vi "General PID Simulator Arduino C code.vi"() -> ()   [LabVIEW 2020]
doc: "This example demonstrates how to simulate a general PID controller."
uses:
  <vilib>/addons/control/pid/NI_PID_pid.lvlib
  <vilib>/addons/control/pid/pid.llb/PID (DBL).vi
panel:
  out "pid_error_integral":dbl=725.9731425642199
  in  "lower limit":dbl
  in  "upper limit":dbl
  in  "Kd":bool=TRUE
  in  "Ki":bool=TRUE
  in  "Kp":bool=TRUE
  in  "loop time[s]":dbl=0.1
  out "PID parameters":dbl[][](graph)=[[30.750899076372775], [7.259731425642199], [0.0]]
  in  "PID type":T1(ring)=enum."Custom C written"
  out "Error":dbl(graph)=1.5375449538186388
  in  "process parameters":T2={"static gain"=2.5, "lag (min)"=18.0, "dead cycles"=0.0, "load %"=40.0, "deadband"=2.0, "noise level %"=0.25, "initial PV"=0.0, "initial PV 2"=0.0}
  out "Manipulated variable":dbl(graph)=38.010630502014976
  in  "SP:":dbl(slide)=88.23529411764706 min=0.0 max=0.0 scale=0.0..100.0
  out "MV:":dbl(slide)=38.010630502014976 scale=-100.0..100.0
  out "PV:":dbl(slide)=86.69774916382842 scale=0.0..100.0
  in  "PID gains":T3={"proportional gain (Kc)"=20.0, "integral time (Ti, min)"=0.01, "derivative time (Td, min)"=0.001} {"derivative time (Td, min)" format="%.3f"; "integral time (Ti, min)" format="%.3f"; "proportional gain (Kc)" format="%.3f"}
  in  "Stop":bool
  out "Process variable and Setpoint":cluster{"initial PV":dbl, "SP:":dbl}(graph)={"initial PV"=86.69774916382842, "SP:"=88.23529411764706}
  # "20,000"
  # "0,008"
  # "0,001"
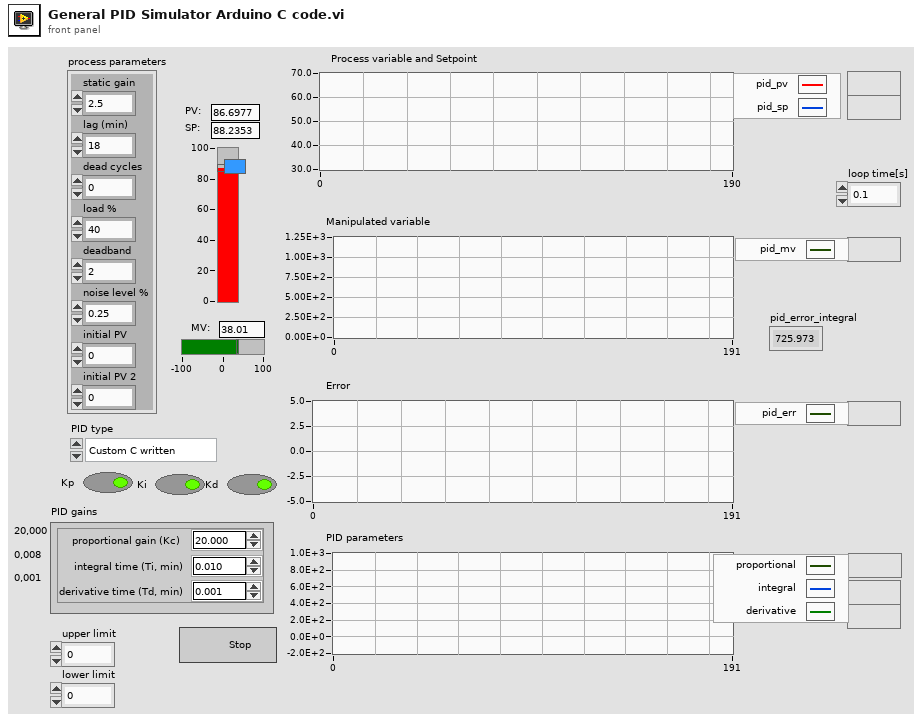
[diagram p1: front panel]
types:
  T1 = enum16{"Official LabVIEW", "Custom LabVIEW", "Custom C written"}
  T2 = cluster{"static gain":dbl, "lag (min)":dbl, "dead cycles":dbl, "load %":dbl, "deadband":dbl, "noise level %":dbl, "initial PV":dbl, "initial PV 2":dbl}
  T3 = cluster{"proportional gain (Kc)":dbl, "integral time (Ti, min)":dbl, "derivative time (Td, min)":dbl}
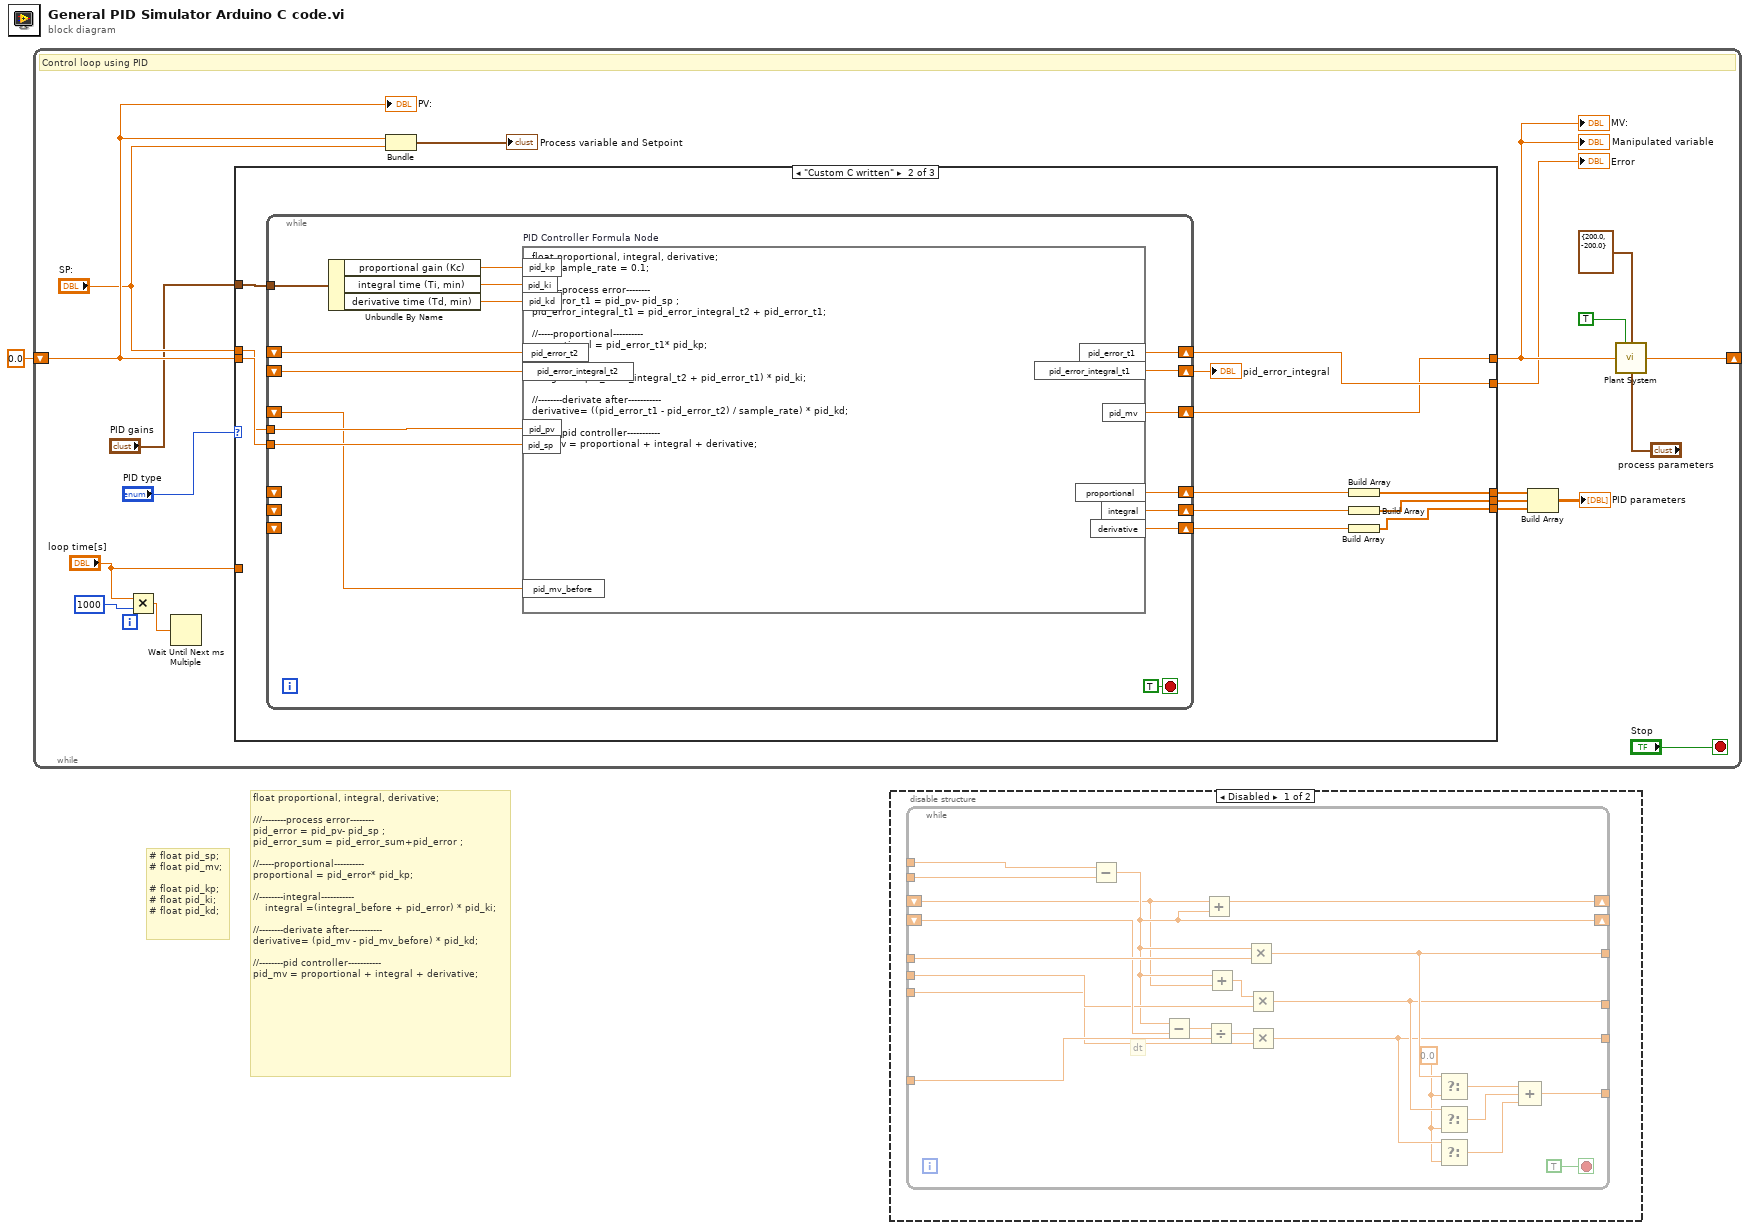
[diagram p0: block diagram]
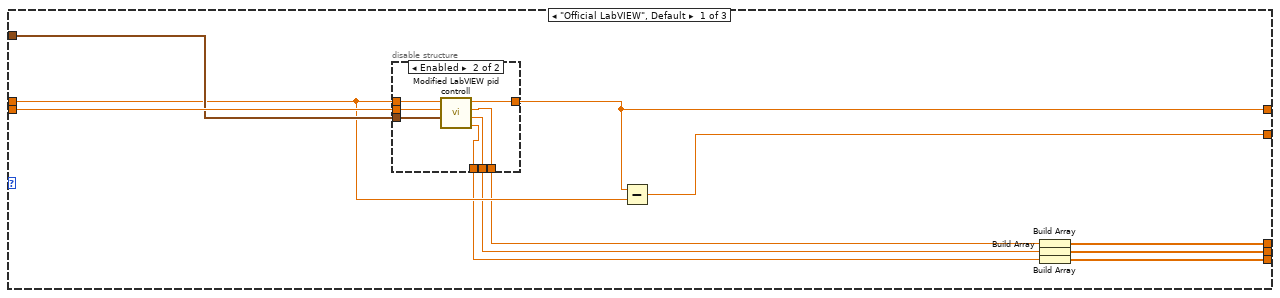
[diagram p3: hidden frame]
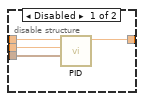
[diagram p4: hidden frame]
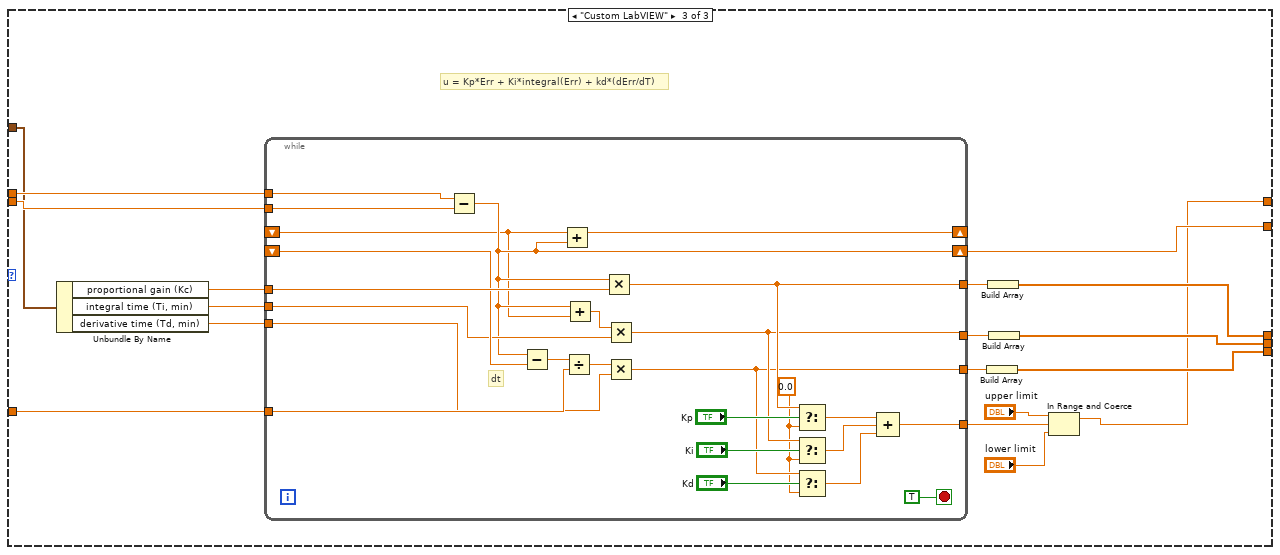
[diagram p5: hidden frame]
diagram:
  # "float proportional, integral, derivative;\n\n///--------process error--------\npid_error = pid_pv- pid_sp ;\npid_error_sum = pid_error_sum+pid_error ;\n\n//-----proportional----------\nproportional = pid_error* pid_kp;\n\n//--------integral-----------\n    integral =(integral_before + pid_error) * pid_ki;\n\n//--------derivate after-----------\nderivative= (pid_mv - pid_mv_before) * pid_kd;\n\n//--------pid controller-----------\npid_mv = proportional + integral + derivative;"
  # "# float pid_sp;\n# float pid_mv;\n\n# float pid_kp;\n# float pid_ki;\n# float pid_kd;"
  n1 = while {
    shift-left: 0.0 ("Plant Output") -> [w18]
    shift-right: [w19] -> _
    stop <- "Stop" stop-if-true
    # "Control loop using PID"
    n2 = Multiply(x="loop time[s]", y=u32 1000) -> (x*y=w2:dbl)
    n3 = Wait Until Next ms Multiple(millisecond multiple=w2) -> ()  [unwired: 1 out]
    n4 = case shown="\"Custom C written\"" "PID type" {
      tunnel: w18 -> [w31 w54 w87]
      tunnel: "SP:" -> [w28 w53 w88]
      tunnel: [w29 w50 w73] -> w15
      tunnel: "PID gains" -> [w30 w52 w85]
      tunnel: [w27 w51 w86] -> w10
      tunnel: [w23 w46 w77] -> w8
      tunnel: [w22 w45 w76] -> w7
      tunnel: [w21 w44 w75] -> w6
      tunnel: "loop time[s]" -> [_ _ w81]
      frame "Official LabVIEW", Default {
        n5 = disable-structure shown="Enabled" {
          disable-tunnel: w31 -> [w35 w41]
          disable-tunnel: w30 -> [w34 w40]
          disable-tunnel: [w33 w39] -> w29
          disable-tunnel: w28 -> [w32 w42]
          disable-tunnel: [_ w38] -> w26
          disable-tunnel: [_ w37] -> w25
          disable-tunnel: [_ w36] -> w24
          frame Disabled {
            n6 = call-poly <vilib>:"PID.vi"("PID gains"=w34, "process variable"=w35, "setpoint"=w32) -> ("output"=w33:dbl)  [unwired: 7 in, 1 out]
          }
          frame Enabled {
            n7 = call "Modified LabVIEW pid controll.vi"("PID gains"=w40, "process variable"=w41, "setpoint"=w42) -> ("derivative"=w36:dbl, "integrated"=w37:dbl, "proportional"=w38:dbl, "output"=w39:dbl)  [unwired: 4 in, 1 out]
          }
        }
        n8 = Subtract(x=w29, y=w28) -> (x-y=w27:dbl)
        n9 = Build Array(w26) -> (w23:dbl[])
        n10 = Build Array(w25) -> (w22:dbl[])
        n11 = Build Array(w24) -> (w21:dbl[])
      }
      frame "Custom C written" {
        n12 = while {
          tunnel: w54 -> [w70]
          tunnel: w53 -> [w69]
          tunnel: w52 -> [w68]
          shift-right: [w62] -> w49
          shift-left: _ -> [_]
          shift-right: [w61] -> w48
          shift-left: _ -> [_]
          shift-right: [w60] -> w47
          shift-left: _ -> [_]
          shift-right: [w63] -> w50
          shift-left: _ -> [w58]
          shift-right: [w67] -> w51
          shift-left: _ -> [w55]
          shift-right: [w57] -> w43
          shift-left: _ -> [w56]
          stop <- TRUE stop-if-true
          n13 = Unbundle By Name(w68) -> ("proportional gain (Kc)"=w66:dbl, "integral time (Ti, min)"=w65:dbl, "derivative time (Td, min)"=w64:dbl)
          n14 = formula code="float proportional, integral, derivative;\nfloat sample_rate = 0.1;\n\n//--------process error--------\npid_error_t1 = pid_pv- pid_sp ;\npid_error_integral_t1 = pid_error_integral_t2 + pid_error_t1;\n\n//-----proportional----------\nproportional = pid_error_t1* pid_kp;\n\n//--------integral-----------\nintegral =(pid_error_integral_t2 + pid_error_t1) * pid_ki;\n\n//--------derivate after-----------\nderivative= ((pid_error_t1 - pid_error_t2) / sample_rate) * pid_kd;\n\n//--------pid controller-----------\npid_mv = proportional + integral + derivative;" "PID Controller Formula Node"("pid_pv"=w69, "pid_sp"=w70, "pid_kp"=w66, "pid_ki"=w65, "pid_kd"=w64, "pid_mv_before"=w58, "pid_error_t2"=w55, "pid_error_integral_t2"=w56) -> ("pid_mv"=w63:dbl, "pid_error_t1"=w67:dbl, "integral"=w61:dbl, "proportional"=w62:dbl, "derivative"=w60:dbl, "pid_error_integral_t1"=w57:dbl)
        }
        "pid_error_integral" <- w43
        n15 = Build Array(w49) -> (w46:dbl[])
        n16 = Build Array(w48) -> (w45:dbl[])
        n17 = Build Array(w47) -> (w44:dbl[])
      }
      frame "Custom LabVIEW" {
        # "u = Kp*Err + Ki*integral(Err) + kd*(dErr/dT)"
        n18 = Unbundle By Name(w85) -> ("proportional gain (Kc)"=w84:dbl, "integral time (Ti, min)"=w83:dbl, "derivative time (Td, min)"=w82:dbl)
        n19 = while {
          tunnel: w88 -> [w112]
          tunnel: w87 -> [w111]
          tunnel: [w110] -> w74
          tunnel: w84 -> [w109]
          tunnel: w83 -> [w103]
          tunnel: w82 -> [w99]
          shift-right: [w102] -> w86
          shift-left: _ -> [w108]
          tunnel: w81 -> [w106]
          shift-right: [w101] -> _
          shift-left: _ -> [w100]
          tunnel: [w93] -> w78
          tunnel: [w94] -> w79
          tunnel: [w95] -> w80
          stop <- TRUE stop-if-true
          w89 = 0.0 ("f")
          # "dt"
          n20 = Subtract(x=w112, y=w111) -> (x-y=w102:dbl)
          n21 = Subtract(x=w102, y=w108) -> (x-y=w107:dbl)
          n22 = Add(x=w100, y=w102) -> (x+y=w101:dbl)
          n23 = Divide(x=w107, y=w106) -> (x/y=w105:dbl)
          n24 = Add(x=w102, y=w100) -> (x+y=w104:dbl)
          n25 = Multiply(x=w102, y=w109) -> (x*y=w95:dbl)
          n26 = Multiply(x=w104, y=w103) -> (x*y=w94:dbl)
          n27 = Multiply(x=w105, y=w99) -> (x*y=w93:dbl)
          n28 = Select(t=w95, s="Kp", f=w89) -> (s? t:f=w92:dbl)
          n29 = Select(t=w94, s="Ki", f=w89) -> (s? t:f=w91:dbl)
          n30 = Select(t=w93, s="Kd", f=w89) -> (s? t:f=w90:dbl)
          n31 = Compound Arithmetic op=ADD(w92, w91, w90) -> (w110:dbl)
        }
        n32 = Build Array(w78) -> (w75:dbl[])
        n33 = Build Array(w80) -> (w77:dbl[])
        n34 = Build Array(w79) -> (w76:dbl[])
        n35 = In Range and Coerce(upper limit="upper limit", x=w74, lower limit="lower limit") -> (coerced(x)=w73:dbl)  [unwired: 1 out]
      }
    }
    "MV:" <- w15
    "Manipulated variable" <- w15
    "Error" <- w10
    n36 = Bundle("Plant Output"=w18, "SP:"="SP:") -> (→"Process variable and Setpoint":cluster{"Plant Output":dbl, "SP:":dbl})  [unwired: 1 in]
    n37 = Build Array(w8, w7, w6) -> (→"PID parameters":dbl[][])
    n38 = call "Plant System.vi"("Integrator ?"=TRUE, "output saturation range"=cluster{"output high":dbl, "output low":dbl} {"output high"=200.0, "output low"=-200.0}, "Plant Input"=w15, "process parameters"="process parameters") -> ("Plant Output"=w19:dbl)  [unwired: 11 in]
    "PV:" <- w18
  }
  n39 = disable-structure shown="Disabled" {
    frame Disabled {
      n40 = while {
        tunnel: _ -> [w137]
        tunnel: _ -> [w136]
        tunnel: [w135] -> _
        tunnel: _ -> [w134]
        tunnel: _ -> [w128]
        tunnel: _ -> [w124]
        shift-right: [w127] -> _
        shift-left: _ -> [w133]
        tunnel: _ -> [w131]
        shift-right: [w126] -> _
        shift-left: _ -> [w125]
        tunnel: [w118] -> _
        tunnel: [w119] -> _
        tunnel: [w120] -> _
        stop <- TRUE stop-if-true
        w114 = 0.0 ("f")
        # "dt"
        n41 = Subtract(x=w137, y=w136) -> (x-y=w127:dbl)
        n42 = Subtract(x=w127, y=w133) -> (x-y=w132:dbl)
        n43 = Add(x=w125, y=w127) -> (x+y=w126:dbl)
        n44 = Divide(x=w132, y=w131) -> (x/y=w130:dbl)
        n45 = Add(x=w127, y=w125) -> (x+y=w129:dbl)
        n46 = Multiply(x=w127, y=w134) -> (x*y=w120:dbl)
        n47 = Multiply(x=w129, y=w128) -> (x*y=w119:dbl)
        n48 = Multiply(x=w130, y=w124) -> (x*y=w118:dbl)
        n49 = Select(t=w120, f=w114) -> (s=w123:bool, s? t:f=w117:dbl)
        n50 = Select(t=w119, f=w114) -> (s=w122:bool, s? t:f=w116:dbl)
        n51 = Select(t=w118, f=w114) -> (s=w121:bool, s? t:f=w115:dbl)
        n52 = Compound Arithmetic op=ADD(w117, w116, w115) -> (w135:dbl)
      }
    }
    frame Enabled {
    }
  }
